vi "Receive.vi"(8 "error in":errorcluster, 11 "framework in":refnum<class "Framework.lvclass">) -> (0 "error out":errorcluster, 3 "framework out":refnum<class "Framework.lvclass">)   [LabVIEW 2019, in "DSF Core.lvlib" / "Framework.lvclass"]
uses:
  Framework.lvclass
  Framework States.ctl
  Framework.lvclass/Framework.ctl
  <vilib>/NI/Memory Manager/Classes/Pointer/Pointer.lvclass/Pointer.ctl
  Pointers/Error/Error Pointer.lvclass/Error Pointer.ctl
  Interface/Interface.lvclass/Interface.ctl
  Performance/Performance.lvclass/Performance.ctl
  Plugin/Plugin.lvclass/Plugin.ctl
  Transfer Group/Transfer Group.lvclass/Transfer Group.ctl
  Timing/Timing.lvclass/Timing.ctl
  Buffers/Buffers.lvclass/Buffers.ctl
  <vilib>/NI/Memory Manager/Classes/Pointer/Write.vi
  <vilib>/NI/Memory Manager/Classes/Pointer/Write U8.vi
  Interface/Logging/Send.vi
  Interface/Logging/Send Logging Command.vi
  Read State.vi
  Pointers/Error/Write Error Pointer.vi
  <vilib>/NI/Memory Manager/Classes/Pointer/Get Address.vi
  <vilib>/NI/Memory Manager/Classes/Pointer/Write (No Check).vi
  <vilib>/NI/Memory Manager/Classes/Pointer/Write (No Check) U8.vi
  <vilib>/NI/Memory Manager/Classes/Pointer/Check Move.vi
  Interface/Send Command.vi
  Interface/Errors.vi
  Interface/Dispatcher/Command Timeout.vi
  <vilib>/NI/Memory Manager/Classes/Pointer/Read.vi
  <vilib>/NI/Memory Manager/Classes/Pointer/Read U8.vi
  <vilib>/NI/Memory Manager/Classes/Pointer/Write 1D U8.vi
  <vilib>/NI/Memory Manager/Classes/Pointer/Clear.vi
  Pointers/Error/Get Power Of 2.vi
  Transfer Group/Increment Iteration.vi
  Thread/Dispatcher/Dispatch Transfer Group.vi
  Transfer Group/Get ID.vi
  Transfer Group/Get Iteration and Late Count.vi
  Plugin/Get ID.vi
  Transfer Group/Copy Async to Inline.vi
  Transfer Group/Wait For Previous.vi
  Transfer Group/Get Active.vi
  <vilib>/NI/Memory Manager/Classes/Pointer/Check Null Pointer.vi
  <vilib>/NI/Memory Manager/Classes/Pointer/Check Count.vi
  <vilib>/NI/Memory Manager/Classes/Pointer/Check Bounds (Power of 2).vi
  Interface/Write RT FIFO.vi
  Interface/New Interface Error.vi
  <vilib>/NI/Memory Manager/Classes/Pointer/Read (No Check).vi
  <vilib>/NI/Memory Manager/Classes/Pointer/Read (No Check) U8.vi
  <vilib>/NI/Memory Manager/Classes/Pointer/Write (No Check) 1D U8.vi
  <vilib>/NI/Memory Manager/Classes/Pointer/Clear (No Check).vi
  <vilib>/NI/Memory Manager/Classes/Pointer/Check Length.vi
  Timing/Increment Iteration.vi
  Interface/Dispatcher/Send Dispatcher Command.vi
  Timing/Get Iteration.vi
  Buffers/Copy Async to Inline.vi
  Transfer Group/Retrieve from FIFO.vi
  Transfer Group/Is Late.vi
  <vilib>/NI/Memory Manager/Classes/Pointer/Errors.vi
  <vilib>/NI/Memory Manager/Classes/Pointer/Null Pointer.vi
  <vilib>/NI/Memory Manager/Classes/Pointer/Is Null.vi
  <vilib>/NI/Memory Manager/Classes/Pointer/Get Size.vi
  <vilib>/NI/Memory Manager/Classes/Pointer/Out of Bounds.vi
  <vilib>/NI/Memory Manager/Classes/Pointer/Check Bounds.vi
  <vilib>/NI/Memory Manager/VIs/New Error Cluster.vi
  <vilib>/NI/Memory Manager/VIs/New Error Cluster (512B).vi
  <vilib>/NI/Memory Manager/VIs/Set Error Code.vi
  <vilib>/NI/Memory Manager/VIs/Set Error Status.vi
  <vilib>/NI/Memory Manager/VIs/Set Error Source.vi
  <vilib>/NI/Memory Manager/VIs/Write String to Source.vi
  Interface/Interface Error Info.vi
  <vilib>/NI/Memory Manager/Classes/Pointer/Check Bounds (Pointer).vi
  Interface/Dispatcher/Write.vi
  Interface/Dispatcher/Write Dispatcher Command.vi
  <vilib>/NI/Memory Manager/Classes/Pointer/Copy All.vi
  Transfer Group/Read Return FIFO.vi
  Transfer Group/Errors.vi
  Transfer Group/Invalid Iteration Error.vi
  Transfer Group/Increment Late Count.vi
  Transfer Group/Return Timeout Error.vi
  <vilib>/NI/Memory Manager/Classes/Pointer/Create Error.vi
  <vilib>/NI/Memory Manager/Classes/Pointer/Write Pointer Size to Error.vi
  <vilib>/NI/Memory Manager/VIs/Write Numeric to Source.vi
  <vilib>/NI/Memory Manager/VIs/Write Numeric Scalar to Source (Base10 U64).vi
  <vilib>/NI/Memory Manager/Classes/Pointer/Check Bounds (Buffer).vi
  VIs/Constants/Constants.vi
  VIs/Constants/Base Error Code.vi
  Interface/Interface Error Offset.vi
  Interface/Dispatcher/Class Name.vi
  <vilib>/NI/Memory Manager/Classes/Pointer/Copy.vi
  VIs/Constants/Engine Library Name.vi
  Transfer Group/Transfer Group Error Info.vi
  <vilib>/NI/Memory Manager/VIs/Write Numeric Scalar to Source (Base10 I32).vi
  <vilib>/NI/Memory Manager/Constants/Constants.vi
  <vilib>/NI/Memory Manager/Constants/Library Name.vi
  <vilib>/NI/Memory Manager/Classes/Pointer/Pointer Error Info.vi
  <vilib>/NI/Memory Manager/Constants/Pointer Class Name.vi
  <vilib>/NI/Memory Manager/Classes/Pointer/Buffer Underflow.vi
  <vilib>/NI/Memory Manager/Classes/Pointer/Copy (No Check).vi
  Transfer Group/Transfer Group Error Offset.vi
  Pointers/Error/Error Pointer.lvclass
  C:/Program Files (x86)/National Instruments/LabVIEW 2019/vi.lib/NI/Memory Manager/Classes/Pointer/Pointer.lvclass
  Interface/Logging/Logging Interface.lvclass
  C:/Dev/GitHub/niveristand-data-sharing-framework-custom-device/Core/Classes/Interface/Interface.lvclass
  Interface/Dispatcher/Dispatcher Interface.lvclass
  Buffer/Buffer.lvclass
  VIs/VI Name.vi
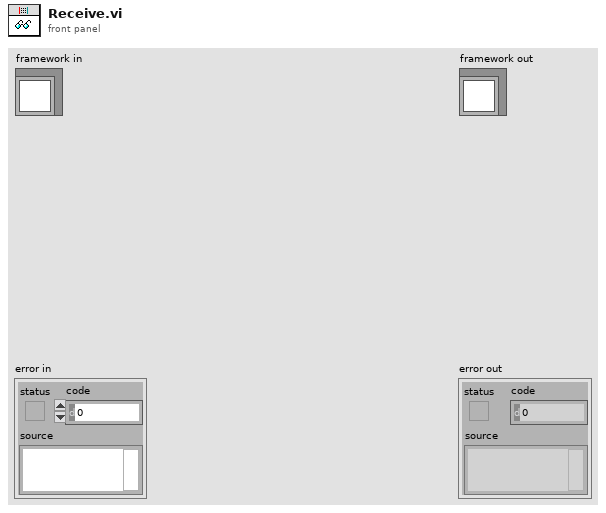
[diagram p1: front panel]
types:
  T1 = typedef "DSF Core.lvlib/Framework.lvclass/Framework States.ctl" = enum8{"Uninitialized", "Initialized", "Start", "Rx", "Tx", "Shutdown"}
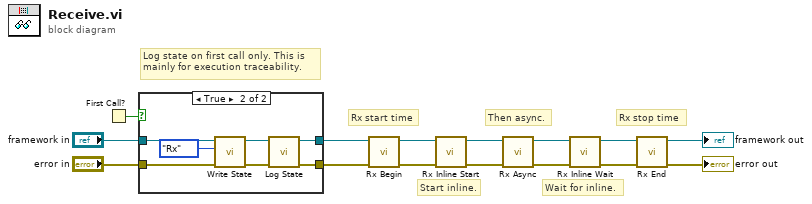
[diagram p0: block diagram]
diagram:
  # "Rx stop time"
  # "Rx start time"
  # "Log state on first call only. This is mainly for execution traceability."
  # "Wait for inline."
  # "Start inline."
  # "Then async."
  n1 = First Call?() -> (First Call?: T/F=w7:bool)
  n2 = case shown="True" w7 {
    tunnel: "error in" -> [w16 w21]
    tunnel: "framework in" -> [w17 w20]
    tunnel: [w16 w19] -> w9
    tunnel: [w17 w18] -> w8
    frame False {
    }
    frame True {
      n3 = call "Write State.vi"("error in (no error)"=w21, "state"=Framework_States."Rx", "Framework in"=w20) -> ("error out"=w22:errorcluster, "Framework out"=w23:refnum<class "Framework.lvclass">)  [unwired: 7 in]
      n4 = call "Log State.vi"("error in (no error)"=w22, "Framework in"=w23) -> ("error out"=w19:errorcluster, "Framework out"=w18:refnum<class "Framework.lvclass">)  [unwired: 8 in]
    }
  }
  n5 = call "Rx Begin.vi"("error in (no error)"=w9, "Framework in"=w8) -> ("error out"=w5:errorcluster, "Framework out"=w6:refnum<class "Framework.lvclass">)  [unwired: 8 in]
  n6 = call "Rx Inline Start.vi"("error in (no error)"=w5, "Framework in"=w6) -> ("error out"=w3:errorcluster, "Framework out"=w4:refnum<class "Framework.lvclass">)  [unwired: 8 in]
  n7 = call "Rx Async.vi"("error in (no error)"=w3, "Framework in"=w4) -> ("error out"=w1:errorcluster, "Framework out"=w2:refnum<class "Framework.lvclass">)  [unwired: 8 in]
  n8 = call "Rx Inline Wait.vi"("error in (no error)"=w1, "Framework in"=w2) -> ("error out"=w13:errorcluster, "Framework out"=w12:refnum<class "Framework.lvclass">)  [unwired: 8 in]
  n9 = call "Rx End.vi"("error in (no error)"=w13, "Framework in"=w12) -> ("error out"=→"error out":errorcluster, "Framework out"=→"framework out":refnum<class "Framework.lvclass">)  [unwired: 8 in]
